vi "Abort Test.vi"() -> ()   [LabVIEW 2020]
uses:
  <instrlib>/BDAQ-6104/Public/Data/Abort Read.vi
panel:
  in  "Abort Read":bool
  in  "Stop":bool
  in  "Abort":bool
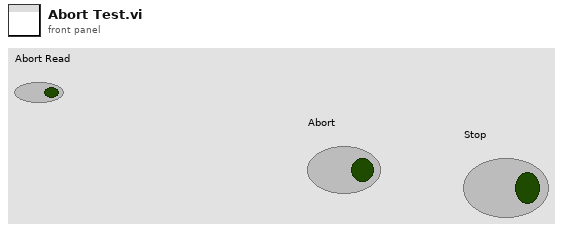
[diagram p1: front panel]
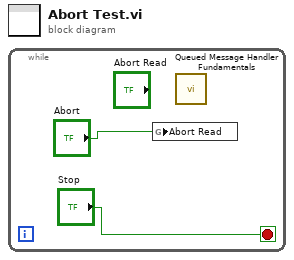
[diagram p0: block diagram]
diagram:
  n1 = while {
    stop <- "Stop" stop-if-true
    n2 = global write "Abort Read.vi" "Abort Read"("Abort") -> ()
    n3 = call <instrlib>:"Queued Message Handler Fundamentals.vi"() -> ()  [unwired: 11 in, 1 out]
  }
